vi "Handle Event.vi"(8 "error in (no error)":errorcluster, 9 "Event Source in":refnum<class "Controller Actor.lvclass">, 10 "Event Data":refnum<class "Event.lvclass">, 11 "Abstract Source Event Handler in":refnum<class "Abstract Event Handler for Controller Actor.lvclass">) -> (0 "error out":errorcluster, 1 "Event Source out":refnum<class "Controller Actor.lvclass">, 3 "Abstract Source Event Handler out":refnum<class "Abstract Event Handler for Controller Actor.lvclass">)   [LabVIEW 2016, in "Event Actors.lvlib" / "Abstract Event Handler for Controller Actor.lvclass"]
uses:
  Abstract Event Handler for Controller Actor.lvclass
  Event/Event.lvclass
  Controller Actor/Controller Actor.lvclass
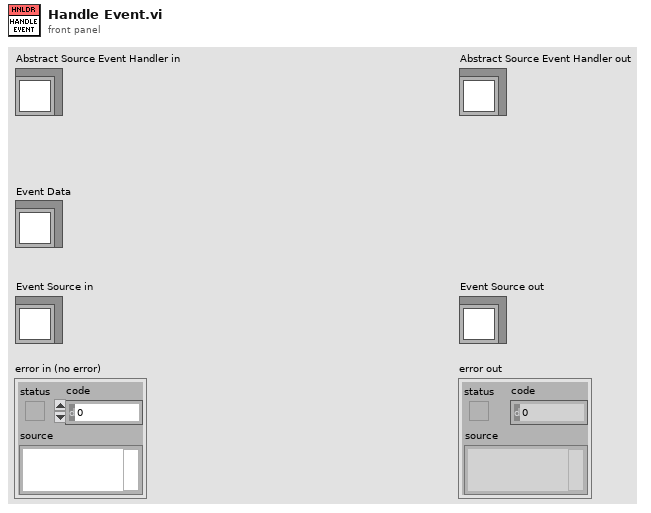
[diagram p1: front panel]
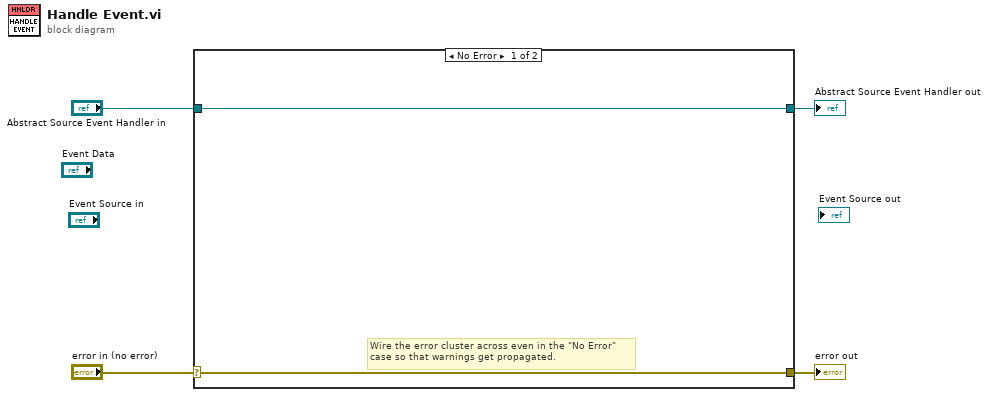
[diagram p0: block diagram]
diagram:
  n1 = case shown="No Error" "error in (no error)" {
    selector: "error in (no error)" -> [w5 w8]
    tunnel: [w5 w8] -> w3
    tunnel: [w6 w7] -> w1
    tunnel: "Abstract Source Event Handler in" -> [w6 w7]
    frame No Error {
      # "Wire the error cluster across even in the \"No Error\"\ncase so that warnings get propagated."
    }
    frame Error {
    }
  }
  "error out" <- w3
  "Abstract Source Event Handler out" <- w1
